vi "LCD Event Based Example.vi"() -> ()   [LabVIEW 2015, in "LabVIEW Interface for Arduino.lvlib"]
doc: "Writes text to the LCD using events to trigger communication when the text changes on the front panel."
uses:
  <vilib>/LabVIEW Interface for Arduino/LabVIEW Interface for Arduino.lvlib
  <vilib>/LabVIEW Interface for Arduino/Type Defs/LCD Pin Config 4 bit.ctl
  <vilib>/LabVIEW Interface for Arduino/Type Defs/Direction.ctl
panel:
  in  "Base (String)":T1(ring)
  in  "LCD Text":string="Hello World"
  in  "Rows":u8=2
  in  "Columns":u8=16
  in  "Stop Button":bool
  in  "LCD Pin Config 4 Bit":T2={"RS"=12, "RW"=255, "Enable"=11, "D4"=5, "D5"=4, "D6"=3, "D7"=2, "LCD"=10}
  # "Configuration"
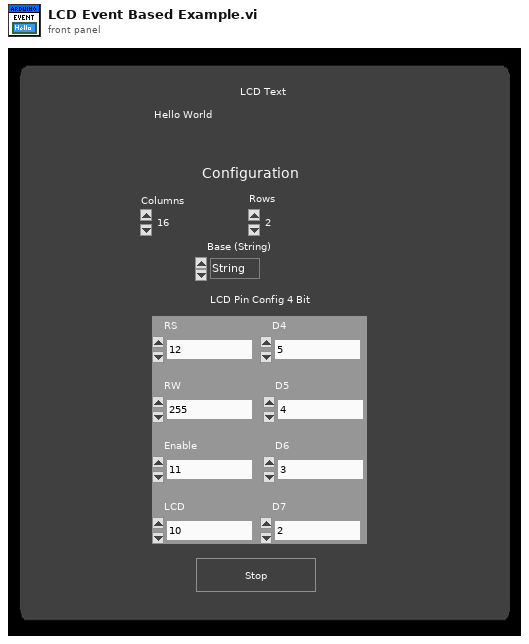
[diagram p1: front panel]
types:
  T1 = enum8{"String", "Binary", "Decimal", "Octal", "Hexadecimal"}
  T2 = typedef "LabVIEW Interface for Arduino.lvlib/LCD Pin Config 4 bit.ctl" = cluster{"RS":u8, "RW":u8, "Enable":u8, "D4":u8, "D5":u8, "D6":u8, "D7":u8, "LCD":u8}
  T3 = typedef "LabVIEW Interface for Arduino.lvlib/Direction.ctl" = enum8{"Left ", "Right"}
  T4 = typedef "LabVIEW Interface for Arduino.lvlib/Arduino Resource.ctl" = cluster{"VISA resource":refnum<visa-resource-name>, "Board Type":T5, "Connection Type":enum8{"USB / Serial"}, "Bytes Per Packet (15)":u8}
  T5 = typedef "LabVIEW Interface for Arduino.lvlib/Board Type.ctl" = enum16{"Uno", "Dimuelanove w/Atmega 328", "Mega 2560"}
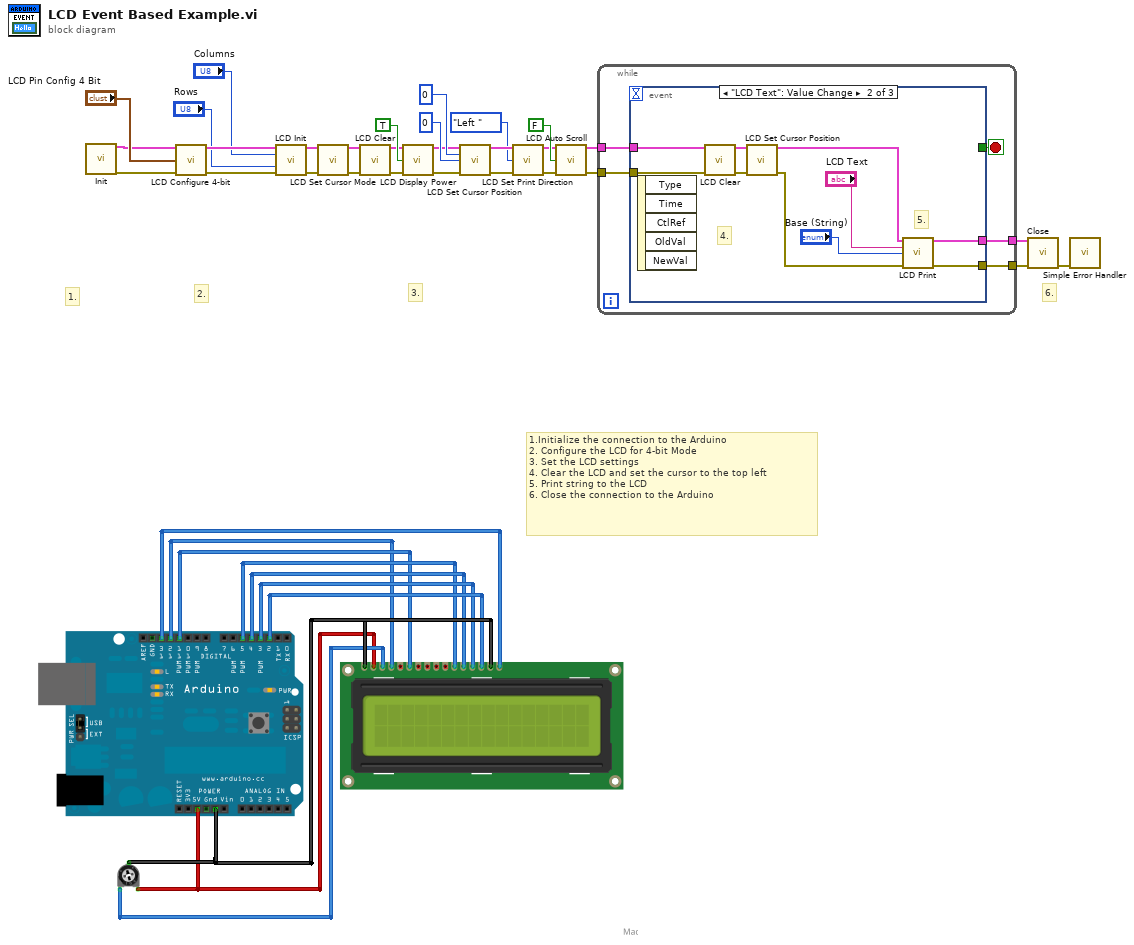
[diagram p0: block diagram]
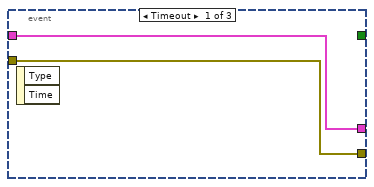
[diagram p2: hidden frame]
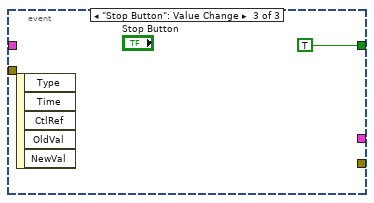
[diagram p3: hidden frame]
diagram:
  # "6."
  # "1.Initialize the connection to the Arduino\n2. Configure the LCD for 4-bit Mode\n3. Set the LCD settings\n4. Clear the LCD and set the cursor to the top left\n5. Print string to the LCD\n6. Close the connection to the Arduino"
  # "3."
  # "2."
  # "1."
  n1 = call <vilib>:"Init.vi"() -> ("Arduino Resource"=w3:T4, "error out"=w5:errorcluster)  [unwired: 18 in]
  n2 = call <vilib>:"LCD Configure 4-bit.vi"("Arduino Resource"=w3, "LCD Pin Config 4 Bit"="LCD Pin Config 4 Bit", "error in"=w5) -> ("Arduino Resource"=w7:T4, "error out"=w6:errorcluster)  [unwired: 11 in]
  n3 = call <vilib>:"LCD Init.vi"("Arduino Resource"=w7, "Columns"="Columns", "Rows"="Rows", "error in"=w6) -> ("Arduino Resource"=w22:T4, "error out"=w21:errorcluster)  [unwired: 10 in]
  n4 = call <vilib>:"LCD Set Cursor Mode.vi"("Arduino Resource"=w22, "error out"=w21) -> ("Arduino Resource"=w20:T4, "error out"=w19:errorcluster)  [unwired: 12 in]
  n5 = call <vilib>:"LCD Clear.vi"("Arduino Resource"=w20, "error in"=w19) -> ("Arduino Resource"=w23:T4, "error out"=w24:errorcluster)  [unwired: 12 in]
  n6 = call <vilib>:"LCD Display Power.vi"("Arduino Resource"=w23, "Display On? (T) 2"=TRUE, "error in"=w24) -> ("Arduino Resource"=w26:T4, "error out"=w27:errorcluster)  [unwired: 11 in]
  n7 = call <vilib>:"LCD Set Cursor Position.vi"("Arduino Resource"=w26, "Column"=u8 0, "Row"=u8 0, "error out"=w27) -> ("Arduino Resource"=w12:T4, "error out"=w11:errorcluster)  [unwired: 10 in]
  n8 = call <vilib>:"LCD Set Print Direction.vi"("Arduino Resource"=w12, "Print Direction"=Direction."Left " ("Direction"), "error in"=w11) -> ("Arduino Resource"=w9:T4, "error"=w8:errorcluster)  [unwired: 11 in]
  n9 = call <vilib>:"LCD Auto Scroll.vi"("Arduino Resource"=w9, "Auto Scroll?"=FALSE ("Auto Scroll? 2"), "error in"=w8) -> ("Arduino Resource"=w15:T4, "error out"=w14:errorcluster)  [unwired: 11 in]
  n10 = while {
    tunnel: w15 -> [w32]
    tunnel: [w34] -> w17
    tunnel: w14 -> [w31]
    tunnel: [w33] -> w16
    stop <- w30 stop-if-true
    n11 = event shown="[1] \"LCD Text\": Value Change" {
      selector: _ -> [_ _ _]
      dyn-events: _ -> [_ _ _]
      timeout: _ -> [_ _ _]
      tunnel: w32 -> [w36 w44 _]
      tunnel: w31 -> [w35 w43 _]
      tunnel: [w36 w46 _] -> w34
      tunnel: [w35 w45 _] -> w33
      tunnel: [_ _ TRUE] -> w30
      event Timeout {
        n12 = event-data() -> ()  [unwired: 1 in, 2 out]
      }
      event "LCD Text": Value Change {
        # "5."
        # "4."
        n13 = event-data() -> ()  [unwired: 1 in, 5 out]
        n14 = call <vilib>:"LCD Clear.vi"("Arduino Resource"=w44, "error in"=w43) -> ("Arduino Resource"=w42:T4, "error out"=w41:errorcluster)  [unwired: 12 in]
        n15 = call <vilib>:"LCD Set Cursor Position.vi"("Arduino Resource"=w42, "error out"=w41) -> ("Arduino Resource"=w40:T4, "error out"=w39:errorcluster)  [unwired: 12 in]
        n16 = call <vilib>:"LCD Print.vi"("Arduino Resource"=w40, "Data"="LCD Text", "Base (String)"="Base (String)", "error out"=w39) -> ("Arduino Resource"=w46:T4, "error out"=w45:errorcluster)  [unwired: 10 in]
      }
      event "Stop Button": Value Change {
        n17 = event-data() -> ()  [unwired: 1 in, 5 out]
      }
    }
  }
  n18 = call <vilib>:"Close.vi"("Arduino Resource"=w17, "error in"=w16) -> ("error out"=w18:errorcluster)  [unwired: 13 in]
  n19 = call <vilib>:"Simple Error Handler.vi"("error in (no error)"=w18) -> ()  [unwired: 4 in, 5 out]
